vi "Search 1D Array of VI References.vi"(1 "start index (0)":i32, 2 "Instance VI Refnum":refnum<vi>, 3 "Connection Process VI RefNums":refnum<vi>[](array[refnum])) -> (0 "index of element":i32)   [LabVIEW 2020, in "JKI TCP Server.lvclass"]
doc: "Searches a 1D array of VI References, <B>by value</B>. This fixes a bug (er... feature) in LabVIEW 8.x where references are searched <B>by object</B> instead of U32 reference value."
uses:
  JKI TCP Server.lvclass
panel:
  # "Copyright © 2004-2008 JKI. All rights reserved.\n\nAuthor: Jim Kring [jim.kring@jameskring.com]\n\nThis library is provided \"AS IS\" ,WITHOUT WARRANTIES OR \nCONDITIONS OF ANY KIND, either express or implied.\n\nJames Kring, Inc. -- http://www.jameskring.com"
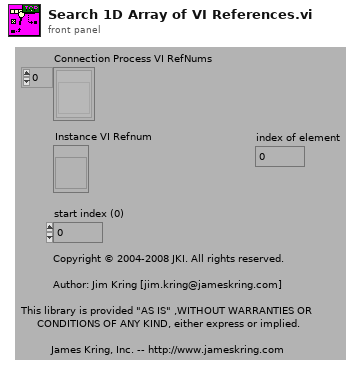
[diagram p1: front panel]
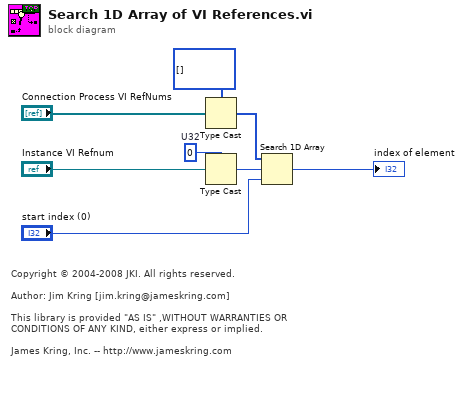
[diagram p0: block diagram]
diagram:
  w1 = u32 0  # U32
  # "Copyright © 2004-2008 JKI. All rights reserved.\n\nAuthor: Jim Kring [jim.kring@jameskring.com]\n\nThis library is provided \"AS IS\" ,WITHOUT WARRANTIES OR \nCONDITIONS OF ANY KIND, either express or implied.\n\nJames Kring, Inc. -- http://www.jameskring.com"
  n1 = Type Cast(type=u32[] [], x="Connection Process VI RefNums") -> (*(type *) &x=w4:u32[])
  n2 = Type Cast(type=w1, x="Instance VI Refnum") -> (*(type *) &x=w2:u32)
  n3 = Search 1D Array(1D array=w4, element=w2, start index (0)="start index (0)") -> (index of element=→"index of element":i32)
